vi "QCP_Get_STR.vi"(0 "QCP Data Block In":T1, 1 "QCP Name":string, 3 "Error In":errorcluster) -> (7 "QCP Data Block Out":T1, 8 "Value Out":string, 10 "Error Out":errorcluster)   [LabVIEW 2015]
uses:
  <userlib>/836-Library/System/QCP Support Code/QCP Data Block.ctl
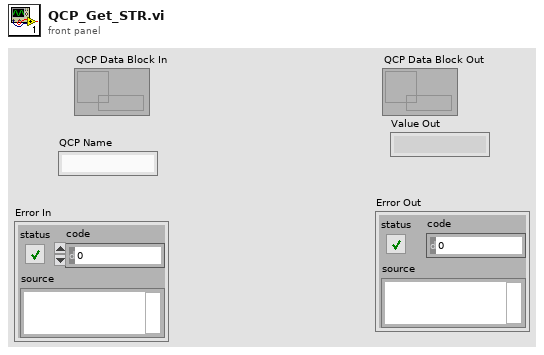
[diagram p1: front panel]
types:
  T1 = typedef "QCP Data Block.ctl" = refnum<data-value>
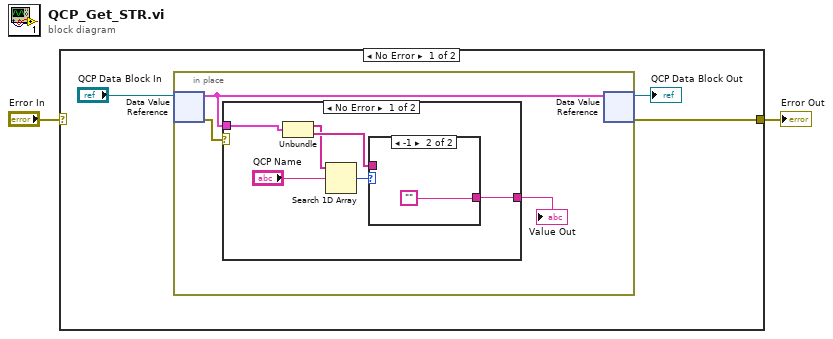
[diagram p0: block diagram]
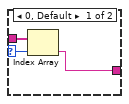
[diagram p2: hidden frame]
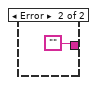
[diagram p3: hidden frame]
diagram:
  n1 = case shown="No Error" "Error In" {
    selector: "Error In" -> [_ w20]
    tunnel: [w5 w20] -> w1
    frame No Error {
      n2 = in-place {
        n3 = in-place-dvr #1("QCP Data Block In") -> (w7:cluster{string[], string[]}, w8:errorcluster)
        n4 = case shown="No Error" w8 {
          tunnel: w7 -> [w10 _]
          tunnel: [w9 ""] -> w6
          frame No Error {
            n5 = Unbundle(w10) -> (w13:string[], w14:string[])
            n6 = Search 1D Array(1D array=w13, element="QCP Name") -> (index of element=w11:i32)  [unwired: 1 out]
            n7 = case shown="-1" w11 {
              selector: w11 -> [w17 _]
              tunnel: [w15 ""] -> w9
              tunnel: w14 -> [w16 _]
              frame 0, Default {
                n8 = Index Array(array=w16, index=w17) -> (element=w15:string)
              }
              frame -1 {
              }
            }
          }
          frame Error {
          }
        }
        "Value Out" <- w6
        n9 = in-place-dvr #1(w7) -> (→"QCP Data Block Out":T1, w5:errorcluster)
      }
    }
    frame Error {
    }
  }
  "Error Out" <- w1
